vi "Generate Wave API.vi"(4 "RX.Data":u8[](array[numeric]), 6 "TX.Data":T1 caption="Transmission Data" format="%.0x", 8 "error in (no error)":errorcluster, 10 "Addr. Mode":refnum<data-value>, 11 "DVR IN":refnum<data-value>) -> (0 "error out":errorcluster, 3 "DVR OUT":refnum<data-value>)   [LabVIEW 2020, in "TX Speed.lvclass"]
uses:
  TX Speed.lvclass
  Addressing Mode/Parent/Addressing Mode.lvclass
  TypeDef/Transmission Data.ctl
  I2C Controller Lib.lvlib
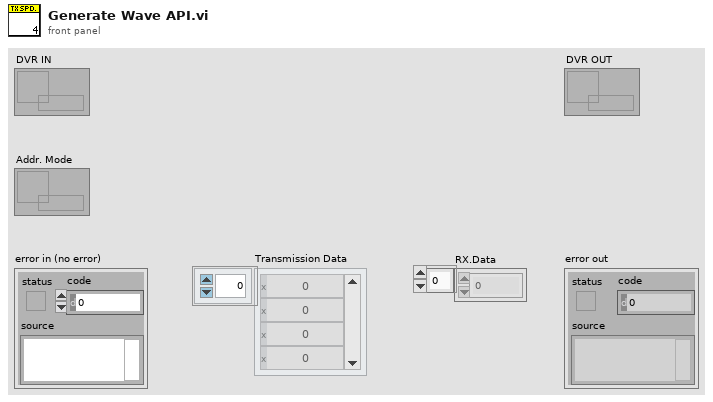
[diagram p1: front panel]
types:
  T1 = typedef "I2C Controller Lib.lvlib/Transmission Data.ctl" = u8[]
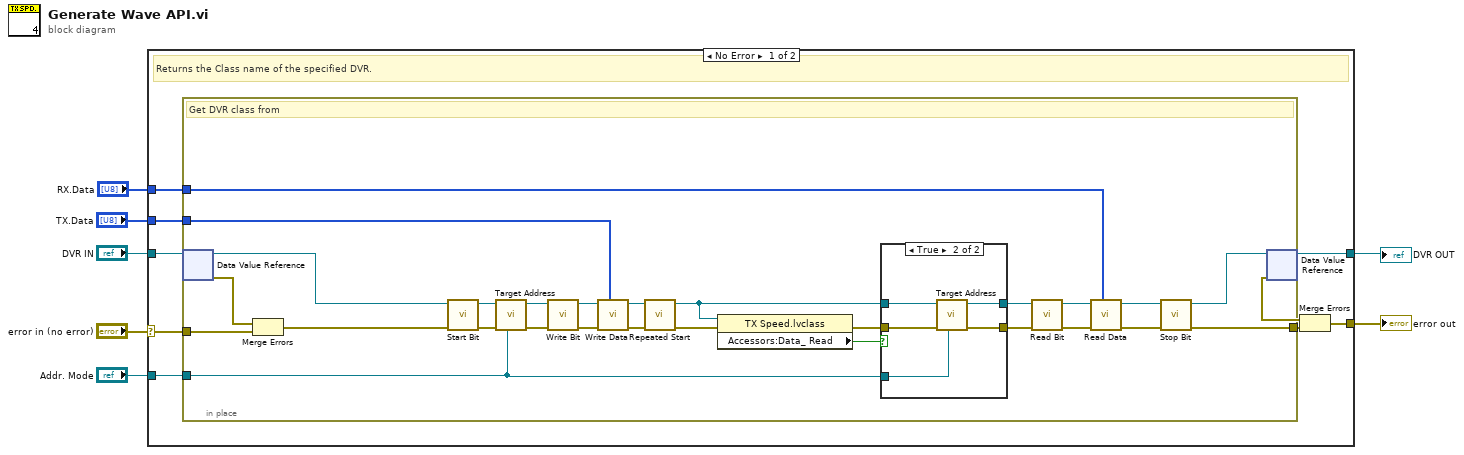
[diagram p0: block diagram]
diagram:
  n1 = case shown="No Error" "error in (no error)" {
    selector: "error in (no error)" -> [w15 w52]
    tunnel: [w16 w51] -> w4
    tunnel: [w13 w52] -> w6
    tunnel: "DVR IN" -> [w10 w51]
    tunnel: "Addr. Mode" -> [w12 _]
    tunnel: "TX.Data" -> [w9 _]
    tunnel: "RX.Data" -> [w8 _]
    frame No Error {
      # "Returns the Class name of the specified DVR."
      n2 = in-place {
        in-place-border: w15 -> [w43]
        in-place-border: w12 -> [w31]
        in-place-border: [w19] -> w11
        in-place-border: w9 -> [w35]
        in-place-border: w8 -> [w34]
        # "Get DVR class from"
        n3 = in-place-dvr #1(w10) -> (w30:refnum<class "TX Speed.lvclass">, w42:errorcluster)
        n4 = Merge Errors(w42, w43) -> (w29:errorcluster)
        n5 = call-dynamic "Start Bit.vi"("error in (no error)"=w29, "TX Speed in"=w30) -> ("error out"=w40:errorcluster, "TX Speed out"=w41:refnum<class "TX Speed.lvclass">)  [unwired: 8 in]
        n6 = call-dynamic "Target Address.vi"("Addr. Mode"=w31, "error in (no error)"=w40, "TX Speed in"=w41) -> ("error out"=w39:errorcluster, "TX Speed out"=w38:refnum<class "TX Speed.lvclass">)  [unwired: 7 in]
        n7 = call-dynamic "Write Bit.vi"("error in (no error)"=w39, "TX Speed in"=w38) -> ("error out"=w36:errorcluster, "TX Speed out"=w37:refnum<class "TX Speed.lvclass">)  [unwired: 8 in]
        n8 = call-dynamic "Write Data.vi"("TX.Data"=w35, "error in (no error)"=w36, "TX Speed in"=w37) -> ("error out"=w33:errorcluster, "TX Speed out"=w32:refnum<class "TX Speed.lvclass">)  [unwired: 7 in]
        n9 = call-dynamic "Repeated Start.vi"("error in (no error)"=w33, "TX Speed in"=w32) -> ("error out"=w24:errorcluster, "TX Speed out"=w22:refnum<class "TX Speed.lvclass">)  [unwired: 8 in]
        n10 = property class="TX Speed.lvclass"(reference=w22, error in=w24) -> (error out=w23:errorcluster, "Accessors:Data_ Read"=w21:bool)  [unwired: 1 out]
        n11 = case shown="True" w21 {
          tunnel: w22 -> [w45 w50]
          tunnel: [w45 w49] -> w26
          tunnel: [w44 w48] -> w25
          tunnel: w31 -> [_ w47]
          tunnel: w23 -> [w44 w46]
          frame False {
          }
          frame True {
            n12 = call-dynamic "Target Address.vi"("Addr. Mode"=w47, "error in (no error)"=w46, "TX Speed in"=w50) -> ("error out"=w48:errorcluster, "TX Speed out"=w49:refnum<class "TX Speed.lvclass">)  [unwired: 7 in]
          }
        }
        n13 = call-dynamic "Read Bit.vi"("error in (no error)"=w25, "TX Speed in"=w26) -> ("error out"=w28:errorcluster, "TX Speed out"=w27:refnum<class "TX Speed.lvclass">)  [unwired: 8 in]
        n14 = call-dynamic "Read Data.vi"("RX.Data"=w34, "error in (no error)"=w28, "TX Speed in"=w27) -> ("error out"=w20:errorcluster, "TX Speed out"=w18:refnum<class "TX Speed.lvclass">)  [unwired: 7 in]
        n15 = call-dynamic "Stop Bit.vi"("error in (no error)"=w20, "TX Speed in"=w18) -> ("error out"=w19:errorcluster, "TX Speed out"=w17:refnum<class "TX Speed.lvclass">)  [unwired: 8 in]
        n16 = in-place-dvr #1(w17) -> (w16:refnum<data-value>, w14:errorcluster)
      }
      n17 = Merge Errors(w14, w11) -> (w13:errorcluster)
    }
    frame Error {
    }
  }
  "error out" <- w6
  "DVR OUT" <- w4
